vi "PmObsCol.vi"(11 "reference":refnum<k24>) -> (2 "Array":refnum<k24>[](array[refnum]))   [LabVIEW 2018, in "Photometrics Camera.lvlib"]
uses:
  Photometrics Camera.lvlib
  C:/FlashGordon/Development/dll/PVCamNET.dll
  Development/dll/PVCamNET.dll
panel:
  out "error out":errorcluster
  in  "error in (no error)":errorcluster
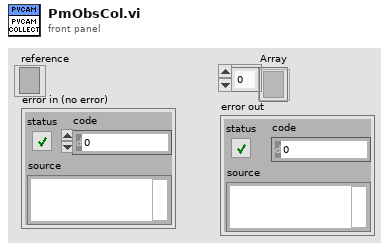
[diagram p1: front panel]
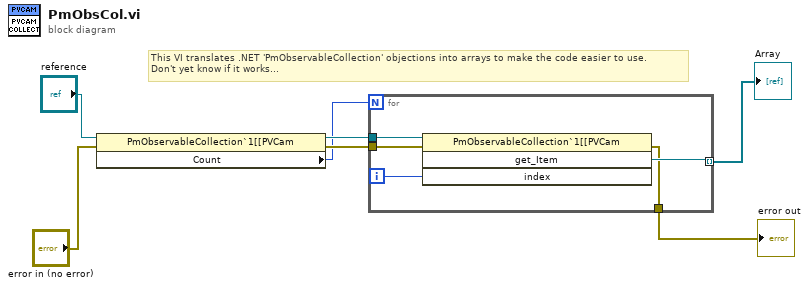
[diagram p0: block diagram]
diagram:
  # "This VI translates .NET 'PmObservableCollection' objections into arrays to make the code easier to use.\nDon't yet know if it works..."
  n1 = property class="PmObservableCollection`1[[PVCam"(reference="reference", error in="error in (no error)") -> (reference out=w6:refnum<k24>, error out=w5:errorcluster, "Count"=w4:i32)
  n2 = for {
    N: w4 -> [_]
    tunnel: w6 -> [w12]
    tunnel: w5 -> [w10]
    tunnel: [w9] -> w3 mode=indexing
    tunnel: [w8] -> w1
    i -> [w11]
    n3 = invoke class="PmObservableCollection`1[[PVCam" method="get_Item"(reference=w12, error in=w10, "index"=w11) -> (error out=w8:errorcluster, "get_Item"=w9:refnum<k24>)  [unwired: 1 in, 2 out]
  }
  "Array" <- w3
  "error out" <- w1
